vi "ReaderCreate.vi"(7 "n_channels":u8, 8 "error in (no error)":errorcluster, 11 "Path":path) -> (0 "error out":errorcluster, 3 "Handle":refnum<data-value>)   [LabVIEW 2020, in "video_io.lvlib"]
uses:
  video_io.lvlib
  common/common.lvlib
  common/bin/gartoolkit_32-1.dll
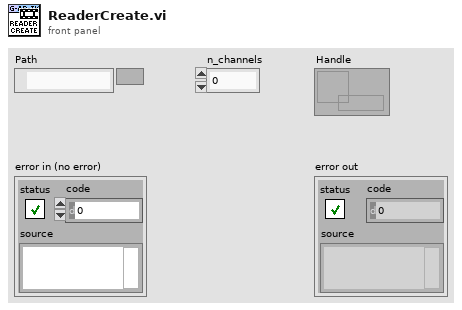
[diagram p1: front panel]
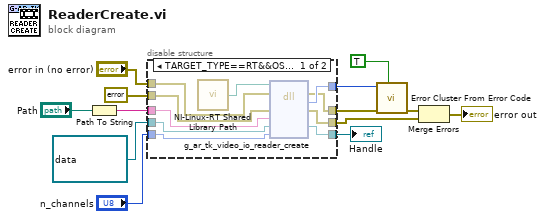
[diagram p0: block diagram]
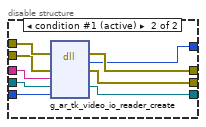
[diagram p2: hidden frame]
diagram:
  n1 = Path To String(path="Path") -> (string=w3:string)
  n2 = disable-structure shown="TARGET_TYPE==RT&&OS==Linux" {
    disable-tunnel: "error in (no error)" -> [w23 w32]
    disable-tunnel: errorcluster {"status"=FALSE, "code"=0, "source"=""} ("error constant") -> [w22 w31]
    disable-tunnel: w3 -> [w21 w25]
    disable-tunnel: refnum<data-value> refnum ("EDVR") -> [w19 w30]
    disable-tunnel: [w15 w29] -> w9
    disable-tunnel: [w17 w28] -> w8
    disable-tunnel: [w16 w27] -> w4
    disable-tunnel: [w14 w26] -> w6
    disable-tunnel: "n_channels" -> [w20 w24]
    frame condition #0 {
      n3 = call "NI-Linux-RT Shared Library Path.vi"() -> ("Path"=w18:path)
      n4 = dll-call lib="?" fn="g_ar_tk_video_io_reader_create" ("g_ar_toolkit.*.*:g_ar_tk_capture_context_create")(path in=w18, error in=w23, "error_cluster"=w22, "Path"=w21, "Handle"=w19, "n_channels"=w20) -> (error out=w15:errorcluster, "return type"=w17:i32, "error_cluster"=w14:errorcluster, "Handle"=w16:refnum<data-value>)  [unwired: 3 in, 1 out]
    }
    frame condition #1 (active) {
      n5 = dll-call lib="C:/serenial/lib/g-augmented-reality-toolkit/LabVIEW/common/bin/gartoolkit_*-1.*" fn="g_ar_tk_video_io_reader_create" ("g_ar_toolkit.*.*:g_ar_tk_capture_context_create")(error in=w32, "error_cluster"=w31, "Path"=w25, "Handle"=w30, "n_channels"=w24) -> (error out=w29:errorcluster, "return type"=w28:i32, "error_cluster"=w26:errorcluster, "Handle"=w27:refnum<data-value>)  [unwired: 4 in, 1 out]
    }
  }
  "Handle" <- w4
  n6 = call <vilib>:"Error Cluster From Error Code.vi"("show call chain? (False)"=TRUE, "error in (no error)"=w9, "error code (0)"=w8) -> ("error out"=w13:errorcluster)  [unwired: 6 in]
  n7 = Merge Errors(w13, w6) -> (→"error out":errorcluster)
